vi "Servo(putinloop).vi"(8 "Count(uSec)":u16=1500, 11 "FPGA I/O Out":refnum<k21>="Port0/DIO0") -> ()   [LabVIEW 2010, in "kevLib2010.lvlib"]
uses:
  kevLib2010.lvlib
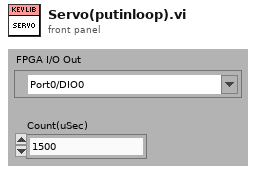
[diagram p1: front panel]
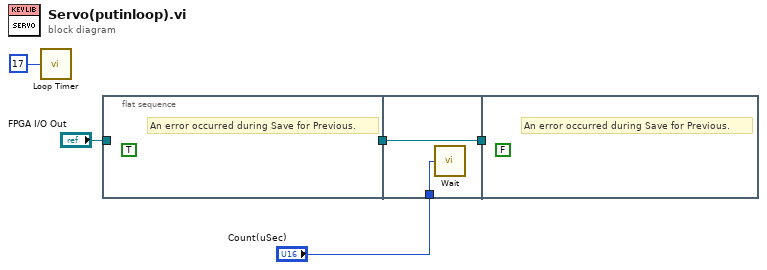
[diagram p0: block diagram]
diagram:
  n1 = call "Loop Timer"("Count(mSec)"=u8 17) -> ()  [unwired: 1 out]
  n2 = flat-sequence {
    tunnel: [_] -> w5
    tunnel: "FPGA I/O Out" -> [w7]
    tunnel: w5 -> [w9]
    tunnel: [w9] -> w4
    tunnel: "Count(uSec)" -> [w8]
    tunnel: w4 -> [_]
    frame #0 {
      w6 = TRUE ("I/O Item")
      # "An error occurred during Save for Previous."
    }
    frame #1 {
      n3 = call "Wait"("Count(uSec)"=w8) -> ()  [unwired: 1 out]
    }
    frame #2 {
      w10 = FALSE ("I/O Item")
      # "An error occurred during Save for Previous."
    }
  }
